vi "Delete Kernel.vi"(8 "Error In":errorcluster, 9 "Kernel In":T1) -> (0 "Error Out":errorcluster)   [LabVIEW 2012]
doc: "Deletes a kernel."
uses:
  Non-User VIs/Controls/Kernel Handle.ctl
  Non-User VIs/Error Checking/Add Error Functional Global.vi
  OpenCLV x64.lvlib
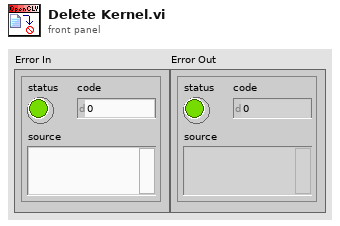
[diagram p1: front panel]
types:
  T1 = typedef "OpenCLV x64.lvlib/Kernel Handle.ctl" = u64
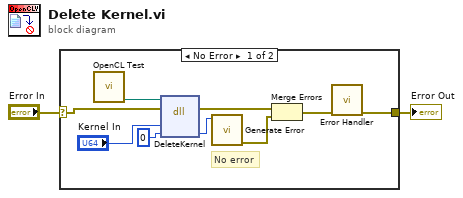
[diagram p0: block diagram]
diagram:
  n1 = case shown="No Error" "Error In" {
    selector: "Error In" -> [w3 w12]
    tunnel: [w7 w12] -> w1
    frame No Error {
      # "No error"
      n2 = call "OpenCL Test.vi"() -> ("DLL To Use"=w8:path)  [unwired: 11 in]
      n3 = dll-call lib="C:/Users/bme-amcelroy-la/Desktop/OpenCLV/trunk/OpenCLV_x64_1.0/OpenCLV_x64.dll" fn="DeleteKernel"(path in=w8, error in=w3, "Kernel In"="Kernel In", "Error"=0) -> (error out=w5:errorcluster, "Error"=w9:i32)  [unwired: 3 in, 1 out]
      n4 = call "Generate Error.vi"("Error"=w9) -> ("error out"=w6:errorcluster)  [unwired: 10 in]
      n5 = Merge Errors(w5, w6) -> (w4:errorcluster)
      n6 = call-poly "Error Handler.vi"("Error In"=w4) -> ("Error Out"=w7:errorcluster)  [unwired: 10 in]
    }
    frame Error {
    }
  }
  "Error Out" <- w1
